vi "RedPitaya_Online_Template_15.12.2019.vi"() -> ()   [LabVIEW 2019]
uses:
  <vilib>/express/express analysis/Spectral/Block/exnSpectralBlock spectral measurements RMS poly.vi
  <vilib>/express/express analysis/Spectral/Block/exnSpectralBlock spectral measurements RMS WFM.vi
  <vilib>/express/express analysis/Spectral/XNode/ExpressSpectralMeasurementsBlockNode.xnode
  <vilib>/Analysis/NI_AAL_SigProc.lvlib
panel:
  in  "Tab Control":T1(tab)
  out "Sensor Signal":sgl[](graph)
  out "Distance [cm]":dbl=113.44243982344857 min=3.0
  out "Location Peaks":dbl[](array[numeric])=[13266.880953082853, 13315.264704454277, 13363.166666666666, 13411.245095976436, 13459.362746922821, 13507.676470231214, 13555.816666494702, 13604.136361362456, 13652.515151704645, 13700.888889844256, 13749.236109598463, 13794.643617108855]
  in  "Peak Threshold":dbl=0.13000000000000012 format="%.2p"
  in  "Sample Threshold":dbl=3000.0 min=3.0
  out "Amplitude Peaks":dbl[](array[numeric])=[1.0525538402918093, 1.1717175096273422, 1.1765014380216599, 1.1719160825014114, 1.1779817342758179, 1.171861931681633, 1.1780178397893906, 1.1718258261680603, 1.1793176233768463, 1.1717897206544876, 1.1821699291467667, 1.171753615140915, 1.184318169951439, 1.1717175096273422, 1.184877797961235, 0.2751458230614705, 1.2100610807538033, 1.1757071167230606, 1.1717175096273422, 1.1720785647630692, 1.1717897206544876, 1.1726201325654984, 1.1720424592494965, 1.176952749490738, 1.1717355698347092, 1.1719521880149841, 1.1719341427087784, 1.175887644290924, 1.1720063537359238, 1.175887644290924, 1.1719521880149841, 1.1751294434070587, 1.1744976043701172, 1.1717716753482819, 1.1717355698347092, 1.1721507757902145, 1.1720063537359238, 1.1727104038000107, 1.1718799769878387, 1.1756890714168549, 1.174901516355678, 1.183162808418274, 1.1716994643211365, 1.1723674088716507, 1.1719521880149841, 1.179714784026146, 1.1716994643211365, 1.1745517551898956, 1.1716994643211365, 1.1733061373233795, 0.621755089566972, 1.171753615140915, 1.1721688210964203, 1.1718258261680603, 1.1855638027191162, 1.1717716753482819, 1.1846972852945328, 1.1933805495500565, 0.9840829961703802, 1.1724576652050018, 1.1742448657751083, 1.1717175096273422, 1.1726381927728653, 1.1718258261680603, 1.1718980371952057, 0.8991820326853672, 0.7123355711971745, 0.3907966132539536, 1.1765375286340714, 1.171970248222351, 1.1716994643211365, 1.1724215596914291, 1.178090050816536, 0.3379421334707791, 0.41264586022121436, 0.14170301344722616, 0.20441930856339144, 0.41122105244403157, 0.1451181683245933, 1.1752962568619767, 1.1743932708955653, 0.956895586745178, 0.2873700125650926, 0.28453465125330124, 0.26024648196001854, 0.22424643172903463, 0.6516108880722223, 0.817807705048344, 0.5987461978823481, 0.20632089172380855, 0.25759756730662464, 0.15722954373967912, 0.39842245914885255, 0.36020466908620663, 0.5011447501881409, 0.40714744730665786, 0.1459626532326326, 0.2610490028596834, 0.2839160048124498, 0.35683245600389685, 0.24854815198521266, 0.21553977557609758, 0.2300543925862896, 0.1404111949016048, 0.13827568641129184, 0.13304504905583056, 0.1480522338098214, 0.20328529691485017, 0.2699936317900817, 0.33758691614384295, 0.39605161937521344, 0.4480722795488725, 0.4914632839585345, 0.5273669232145075, 0.5538165781670914, 0.5719683082015473, 0.5797038517122126, 0.5348972490031214]
  out "Peaks Detected":i32=118
  in  "Width":i32=3 min=3
  in  "Peaks/Valleys":enum32{"Peaks", "Valleys"}(ring)
  out "Reflection":sgl[](graph)=[-0.027295426, -0.027728686, -0.028017526, -0.027439846, -0.027873106, -0.028306367, -0.028595207, -0.028450787, -0.029028468, -0.028884048, -0.027439846, -0.027584266, -0.027728686, -0.027584266, -0.027295426, -0.028161947, -0.027728686, -0.027873106, -0.027728686, -0.027295426, -0.026862165, -0.027151005, -0.028306367, -0.028595207, -0.029172888, -0.028595207, -0.027728686, -0.027439846, -0.027439846, -0.027295426, -0.027295426, -0.027584266, -0.028017526, -0.028306367, -0.029028468, -0.028884048, -0.028161947, -0.028450787, -0.028884048, -0.028884048, -0.028739627, -0.028450787, -0.028306367, -0.028595207, -0.027873106, -0.028017526, -0.028017526, -0.027728686, -0.028884048, -0.029606149, -0.029317308, -0.028161947, -0.027584266, -0.027584266, -0.028450787, -0.028450787, -0.027728686, -0.028161947, -0.028017526, -0.027584266, -0.028161947, -0.027439846, -0.027151005, -0.027584266, -0.027873106, -0.027728686, -0.028017526, -0.028739627, -0.028161947, -0.027873106, -0.028017526, -0.027584266, -0.027295426, -0.027439846, -0.027728686, -0.028450787, -0.028017526, -0.028450787, -0.027873106, -0.027728686, -0.027439846, -0.027728686, -0.028017526, -0.028017526, -0.028884048, -0.028739627, -0.028739627, -0.028595207, -0.028739627, -0.029028468, -0.028739627, -0.028306367, -0.028306367, -0.028739627, -0.028884048, -0.028595207, -0.028595207, -0.028595207, -0.027151005, -0.027728686, -0.028306367, -0.028595207, -0.027873106, -0.028161947, -0.028017526, -0.027584266, -0.028595207, -0.028595207, -0.027728686, -0.027873106, -0.027295426, -0.027728686, -0.028161947, -0.027873106, -0.027873106, -0.027584266, -0.027873106, -0.027439846, -0.027439846, -0.027873106, -0.027295426, -0.026573325, -0.027006585, -0.028161947, -0.028017526, -0.028306367, -0.029317308, -0.027728686, -0.027873106, -0.027584266, -0.028306367, -0.028161947, -0.028884048, -0.029750569, -0.028595207, -0.028739627, -0.028884048, -0.028161947, -0.027728686, -0.027439846, -0.027728686, -0.027873106, -0.028450787, -0.028739627, -0.029028468, -0.029461728, -0.029028468, -0.028161947, -0.027584266, -0.026573325, -0.027584266, -0.028450787, -0.028450787, -0.027873106, -0.028161947, -0.028017526, -0.027584266, -0.027584266, -0.027006585, -0.026140064, -0.026573325, -0.026862165, -0.027295426, -0.027151005, -0.027295426, -0.028017526, -0.028161947, -0.028017526, -0.027873106, -0.028450787, -0.028739627, -0.028739627, -0.029461728, -0.029172888, -0.028450787, -0.029028468, -0.03003941, -0.03047267, -0.03047267, -0.029750569, -0.028450787, -0.028161947, -0.028739627, -0.028017526, -0.028161947, -0.028161947, -0.028017526, -0.027728686, -0.027006585, -0.026862165, -0.027006585, -0.027295426, -0.027151005, -0.026140064, -0.026284484, -0.026573325, -0.026284484, -0.025562381, -0.0249847, -0.0249847, -0.02484028, -0.025851222, -0.025851222, -0.026140064, -0.026428904, -0.026140064, -0.026573325, -0.027584266, -0.028161947, -0.028017526, -0.028595207, -0.029606149, -0.029606149, -0.03133919, -0.031772453, -0.031483613, -0.03191687, -0.032205712, -0.032638974, -0.032494552, -0.032205712, -0.032350134, -0.031772453, -0.03090593, -0.03090593, -0.029606149, -0.028739627, -0.028595207, -0.028450787, -0.027151005, -0.026140064, -0.0249847, -0.023540499, -0.022673978, -0.021518616, -0.020796515, -0.019641152, -0.01906347, -0.019207891, -0.019641152, -0.019785572, -0.019207891, -0.019352311, -0.020218834, -0.020363254, -0.021374196, -0.022673978, -0.02397376, -0.025562381, -0.027584266, -0.029028468, -0.029750569, -0.03133919, -0.033505496, -0.034660857, -0.03538296, -0.03653832, -0.036827162, -0.037404843, -0.038704623, -0.039426725, -0.039426725, -0.040148824, -0.04043767, -0.039859984, -0.038849045, -0.03812694, -0.03697158, -0.035238538, -0.033794336, -0.032205712, -0.03003941, -0.028161947, -0.025562381, -0.022385137, -0.020074412, -0.016897168, -0.014586444, -0.013575503, -0.013142242, -0.010542678, -0.0088096345, -0.007221012, -0.0069321715, -0.0064989105, -0.00621007, -0.0064989105, -0.007943113, -0.009676156, -0.01242014, -0.014586444, -0.017474849, -0.020218834, -0.023684919, -0.026428904, -0.029750569, -0.033361074, -0.03668274, -0.039426725, -0.04245955, -0.044914693, -0.04794752, -0.050691504, -0.053002227, -0.055457372, -0.056323893, -0.05589063, -0.05617947, -0.05589063, -0.055457372, -0.05430201, -0.051558025, -0.04910288, -0.044481434, -0.040582087, -0.03697158, -0.032638974, -0.028161947, -0.02397376, -0.01906347, -0.012997821, -0.0077986927, -0.0037549261, 0.00043326072, 0.0040437668, 0.0067877513, 0.009242895, 0.011698039, 0.013719923, 0.013864343, 0.01242014, 0.010975938, 0.009242895, 0.0070765917, 0.003610506, -0.00086652144, -0.005343549, -0.010831518, -0.016463907, -0.022240717, -0.027873106, -0.034516435, -0.04043767, -0.046214476, -0.051991284, -0.057334833, -0.063400485, -0.06802193, -0.07293222, -0.07654273, -0.07842019, -0.080730915, -0.08145302, -0.08000881, -0.07899787, -0.076831564, -0.07452084, -0.069899395, -0.06426701, -0.058634616, -0.051558025, -0.045059115, -0.037116002, -0.029028468, -0.020796515, -0.012997821, -0.0056323893, 0.0027439846, 0.010542678, 0.016897168, 0.022673978, 0.028306367, 0.032494552, 0.03538296, 0.03697158, 0.037982523, 0.037693683, 0.035238538, 0.032494552, 0.028161947, 0.022818398, 0.015741806, 0.010253837, 0.0023107238, -0.0056323893, -0.014586444, -0.02397376, -0.034083176, -0.044192594, -0.053579908, -0.06253396, -0.07105476, -0.07914229, -0.0870854, -0.09343989, -0.099072285, -0.10239395, -0.10542677, -0.108170755, -0.1091817, -0.107159816, -0.10369373, -0.09878344, -0.092573375, -0.08593004, -0.07755367, -0.06917729, -0.058056936, -0.04809194, -0.037116002, -0.025273541, -0.013864343, -0.002455144, 0.008665214, 0.019496731, 0.03003941, 0.039571144, 0.04751426, 0.05415759, 0.059501138, 0.062822804, 0.06542237, 0.06672215, 0.06571121, 0.06311164, 0.058345776, 0.052713387, 0.045347955, 0.036827162, 0.027006585, 0.016463907, 0.0046214475, -0.0064989105, -0.01891905, -0.032494552, -0.0463589, -0.06094534, -0.07437642, -0.08679657, -0.09820576, -0.108748436, -0.11755808, -0.12535676, -0.13171126, -0.13589944, -0.13821016, -0.13821016, -0.13676597, -0.13329989, -0.12867843, -0.122323945, -0.113514304, -0.10354931, -0.09228453, -0.07943113, -0.065566786, -0.050980344, -0.03480528, -0.017474849, -0.0012997822, 0.013864343, 0.028739627, 0.04245955, 0.05560179, 0.06816635, 0.07856461, 0.088240765, 0.095172934, 0.0999388, 0.102249525, 0.10311605, 0.101671845, 0.09748366, 0.09112917, 0.082897216, 0.07264338, 0.06123418, 0.04765868, 0.032927815, 0.015886227, -0.0014442024, -0.019785572, -0.0378381, -0.055746213, -0.07379874, -0.09343989, -0.109903805, -0.12521234, -0.13878785, -0.1499082, -0.16016205, -0.16868284, -0.1748929, -0.17835899, -0.1798032, -0.17807016, -0.17330429, -0.16651653, -0.1569848, -0.14586444, -0.1320001, -0.11568061, -0.09791692, -0.07928671, -0.05935672, -0.038271364, -0.017041588, 0.004910288, 0.025706802, 0.045059115, 0.06383374, 0.082319535, 0.09863903, 0.113514304, 0.12550119, 0.13546619, 0.1426872, 0.14687538, 0.14803074, 0.14615329, 0.14080973, 0.13243335, 0.12189068, 0.10961496, 0.093151055, 0.074809685, 0.05560179, 0.034372017, 0.011409199, -0.011264779, -0.0363939, -0.062245123, -0.0870854, -0.10932612, -0.1320001, -0.1535187, -0.17214893, -0.18861283, -0.20233275, -0.2147529, -0.22298485, -0.22789514, -0.23006144, -0.22789514, -0.22298485, -0.21489732, -0.20305486, -0.18861283, -0.1698382, -0.14947495, -0.12622328, -0.101238586, -0.07553179, -0.04823636, -0.020652095, 0.0063544903, 0.033505496, 0.06181186, 0.088818446, 0.11380315, 0.13575502, 0.15496291, 0.17186008, 0.18529117, 0.19511174, 0.20132181, 0.20319928, 0.2026216, 0.19785573, 0.18731305, 0.17431523, 0.15814017, 0.13792133, 0.11481409, 0.08896287, 0.06051208, 0.03105035, 0.00014442024, -0.032061294, -0.064411424, -0.09820576, -0.12968938, -0.1591511, -0.18615769, -0.21186449, -0.23482731, -0.25360194, -0.2690549, -0.28104177, -0.28941816, -0.292451, -0.2905735, -0.28494114, -0.27454287, -0.25880107, -0.2404597, -0.21821898, -0.19222334, -0.16348371, -0.13185568, -0.09835018, -0.06311164, -0.026284484, 0.010253837, 0.04722542, 0.08304164, 0.11596945, 0.1477419, 0.17734805, 0.20392138, 0.22544, 0.24349253, 0.25721243, 0.26645535, 0.26992142, 0.2681884, 0.2618339, 0.24984701, 0.23352753, 0.21287543, 0.18803515, 0.15900669, 0.12737866, 0.09185127, 0.05372433, 0.013719923, -0.028450787, -0.069899395, -0.11105917, -0.15005262, -0.18817957, -0.22471789, -0.25750127, -0.2853744, -0.3103591, -0.33043352, -0.3454532, -0.35498494, -0.35873988, -0.35772893, -0.3503635, -0.3375101, -0.31945756, -0.29707244, -0.2691993, -0.23742688, -0.20103297, -0.16117299, -0.119002275, -0.07610947, -0.03133919, 0.014297604, 0.06022324, 0.10470467, 0.14730865, 0.18687978, 0.22226274, 0.25287983, 0.28104177, 0.30342692, 0.3197464, 0.3318777, 0.3373657, 0.3354882, 0.32725626, 0.31295866, 0.29317307, 0.2690549, 0.23887107, 0.20305486, 0.16333929, 0.12044648, 0.07466526, 0.026717745, -0.023251658, -0.074232005, -0.12304604, -0.17027146, -0.21663035, -0.25923434, -0.29808336, -0.33346632, -0.36379457, -0.3873351, -0.40495434, -0.4175189, -0.42358455, -0.42214036, -0.4140528, -0.39903313, -0.37852544, -0.3518077, -0.3190243, -0.2804641, -0.2375713, -0.19077913, -0.14182067, -0.09084033, -0.03754926, 0.016319487, 0.07004382, 0.12030206, 0.16998263, 0.21648593, 0.25952315, 0.2982278, 0.32985583, 0.35556263, 0.37549263, 0.38921255, 0.39556703, 0.3945561, 0.38632414, 0.37101558, 0.34906372, 0.32075736, 0.28638533, 0.2462365, 0.2004553, 0.15048589, 0.09748366, 0.04231513, -0.014297604, -0.07192128, -0.12766749, -0.18240276, -0.23540498, -0.28522998, -0.3311556, -0.37217095, -0.40668738, -0.43571585, -0.458101, -0.47254303, -0.4788975, -0.47788656, -0.4689325, -0.4531907, -0.4303723, -0.40047732, -0.3632169, -0.32003525, -0.272521, -0.22226274, -0.16810516, -0.10961496, -0.050691504, 0.010253837, 0.07119918, 0.12867843, 0.18456906, 0.23699361, 0.28494114, 0.32855603, 0.36668298, 0.39773333, 0.4211294, 0.43730447, 0.44582528, 0.4475583, 0.4394708, 0.42358455, 0.39946637, 0.36942697, 0.33231097, 0.28884047, 0.23915991, 0.18558, 0.12795633, 0.06672215, 0.004188187, -0.05877904, -0.12304604, -0.18370254, -0.2433481, -0.30024967, -0.35281864, -0.39859986, -0.43802658, -0.47052112, -0.49651676, -0.5147137, -0.52568966, -0.5284337, -0.5216459, -0.5066262, -0.482508, -0.45073557, -0.41260862, -0.36668298, -0.3154138, -0.25923434, -0.19944435, -0.13618828, -0.07119918, -0.0056323893, 0.06094534, 0.124923505, 0.18716863, 0.24681419, 0.30198273, 0.34993023, 0.39311188, 0.42849484, 0.45622352, 0.47702006, 0.48857367, 0.49131766, 0.48539641, 0.4709544, 0.44856927, 0.41708565, 0.37866986, 0.33288866, 0.28075296, 0.22356252, 0.16189508, 0.09676156, 0.029750569, -0.039137885, -0.1084596, -0.17518175, -0.24074854, -0.30357134, -0.36047292, -0.41231978, -0.45795658, -0.49651676, -0.5274227, -0.5500967, -0.5632389, -0.56713825, -0.56266123, -0.549519, -0.52814484, -0.4968056, -0.45781216, -0.4118865, -0.3581622, -0.29938316, -0.2361271, -0.16882727, -0.0999388, -0.029317308, 0.04260397, 0.112503365, 0.18009204, 0.24450347, 0.3048711, 0.3597508, 0.4087093, 0.4495802, 0.48178592, 0.5059041, 0.52121264, 0.5272783, 0.5238122, 0.51196975, 0.49073997, 0.45983404, 0.4211294, 0.37592587, 0.3224904, 0.26313367, 0.19843341, 0.13026705, 0.059212297, -0.013142242, -0.087663084, -0.15929553, -0.22991702, -0.29736128, -0.35989523, -0.41694123, -0.46792158, -0.5109588, -0.5459085, -0.57277066, -0.591112, -0.5997772, -0.59818864, -0.58692384, -0.5662718, -0.53551024, -0.49767214, -0.45116884, -0.3975889, -0.33765453, -0.27223215, -0.20291044, -0.12968938, -0.05516853, 0.01877463, 0.093728736, 0.16593885, 0.23468289, 0.29996082, 0.35902873, 0.41203094, 0.4573789, 0.4946393, 0.5229457, 0.5427312, 0.5525518, 0.5526962, 0.5433089, 0.524101, 0.49536142, 0.458101, 0.4124642, 0.35946196, 0.299672, 0.23482731, 0.16463907, 0.09141801, 0.016030647, -0.06007882, -0.13662155, -0.21114239, -0.2832081, -0.35094118, -0.4124642, -0.4673439, -0.51442486, -0.5544293, -0.5859129, -0.6071427, -0.6184075, -0.621007, -0.61320835, -0.5951558, -0.5675715, -0.5310332, -0.4859741, -0.43282744, -0.3731819, -0.30862606, -0.23742688, -0.16247277, -0.086074464, -0.009387315, 0.06859961, 0.14369814, 0.2176413, 0.28667417, 0.3497858, 0.40654296, 0.45607913, 0.49752772, 0.5307444, 0.5542849, 0.56786036, 0.5719041, 0.5655497, 0.54908574, 0.52251244, 0.4881404, 0.4438034, 0.39224535, 0.3338996, 0.26862165, 0.19814457, 0.12304604, 0.046792157, -0.031483613, -0.110481486, -0.18731305, -0.2619783, -0.33259982, -0.39787775, -0.45636794, -0.5073483, -0.55168533, -0.5875015, -0.61306393, -0.6289501, -0.6344381, -0.6295278, -0.6145081, -0.5901011, -0.55674005, -0.5142805, -0.4630113, -0.40394342, -0.33794335, -0.267033, -0.19308986, -0.116980396, -0.038849045, 0.04072651, 0.11856902, 0.19366755, 0.26529998, 0.33216655, 0.39238977, 0.44640297, 0.4916065, 0.5277116, 0.55414045, 0.5717597, 0.579414, 0.57667, 0.56338334, 0.54056495, 0.5086481, 0.46705505, 0.4167968, 0.36003965, 0.29562822, 0.22500673, 0.15164125, 0.07408758, -0.004332607, -0.08376374, -0.16088414, -0.23742688, -0.30949256, -0.37708125, -0.4388931, -0.49348396, -0.5408538, -0.5792696, -0.6080092, -0.62692827, -0.6355935, -0.6338604, -0.6228845, -0.602088, -0.5706044, -0.5301667, -0.48135266, -0.4245955, -0.36148384, -0.29259542, -0.22038528, -0.14427581, -0.06600005, 0.012997821, 0.09141801, 0.16738306, 0.2397376, 0.30790395, 0.37072676, 0.42632854, 0.47355396, 0.512403, 0.5280004, 0.43499374, 0.34559762, 0.27959758, 0.22933933, 0.19020145, 0.15727364, 0.12925611, 0.10586003, 0.083908156, 0.06311164, 0.04274839, 0.022529557, 0.0021663036, -0.01776369, -0.037693683, -0.057190415, -0.07827577, -0.10326047, -0.115825035, -0.1283896, -0.13979879, -0.15019704, -0.15972878, -0.16680537, -0.17171566, -0.17431523, -0.17518175, -0.17373754, -0.16853842, -0.16102856, -0.15164125, -0.14037648, -0.12622328, -0.110914744, -0.09502852, -0.07813135, -0.0599344, -0.04159303, -0.022529557, -0.0025995644, 0.015164125, 0.032638974, 0.049824983, 0.06513353, 0.08694098, 0.09748366, 0.10412699, 0.10975938, 0.11380315, 0.11654713, 0.11669155, 0.11481409, 0.1106259, 0.10369373, 0.09546178, 0.084197, 0.070477076, 0.056035053, 0.040293247, 0.023107238, 0.0056323893, -0.01242014, -0.03076151, -0.050113823, -0.06816635, -0.09228453, -0.10975938, -0.122757204, -0.1334443, -0.14413139, -0.1535187, -0.16001762, -0.16565001, -0.16882727, -0.17012703, -0.16940494, -0.16536117, -0.15900669, -0.15048589, -0.14052089, -0.12810075, -0.11438083, -0.09878344, -0.0820307, -0.064411424, -0.046503317, -0.028739627, -0.010831518, 0.0075098523, 0.02484028, 0.041448608, 0.056612734, 0.0713436, 0.090407066, 0.0970504, 0.10239395, 0.10744866, 0.11077032, 0.111348, 0.11004822, 0.106148876, 0.100083224, 0.091995694, 0.08217511, 0.07076592, 0.057768095, 0.04318165, 0.027728686, 0.010542678, -0.0069321715, -0.02512912, -0.043037232, -0.06108976, -0.08000881, -0.10268279, -0.11322547, -0.124345824, -0.13561061, -0.1448535, -0.15308546, -0.15900669, -0.16218393, -0.16362813, -0.16377255, -0.16045089, -0.15539618, -0.14788632, -0.13878785, -0.12824517, -0.11568061, -0.10152743, -0.08621888, -0.06946614, -0.051991284, -0.034516435, -0.017186008, -0.00086652144, 0.015741806, 0.031483613, 0.0463589, 0.06036766, 0.07654273, 0.088818446, 0.094161995, 0.09878344, 0.102249525, 0.10412699, 0.10297163, 0.10022765, 0.0948841, 0.08838519, 0.080153234, 0.06975497, 0.057623673, 0.044192594, 0.029461728, 0.014008763, -0.0014442024, -0.01776369, -0.0356718, -0.05256897, -0.06859961, -0.09011823, -0.10484909, -0.11524735, -0.12535676, -0.1348885, -0.14297603, -0.14860843, -0.15250777, -0.15467407, -0.15510733, -0.1535187, -0.14904168, -0.14254278, -0.13445525, -0.12506792, -0.11423641, -0.101238586, -0.08751866, -0.07235454, -0.05617947, -0.04043767, -0.02469586, -0.008665214, 0.0069321715, 0.022240717, 0.03726042, 0.05025824, 0.06152302, 0.076398306, 0.08737425, 0.09069591, 0.093584314, 0.09459525, 0.09445084, 0.09286221, 0.08896287, 0.083908156, 0.07668715, 0.06744425, 0.056323893, 0.044192594, 0.03032825, 0.016463907, 0.0011553619, -0.015164125, -0.03119477, -0.046214476, -0.06094534, -0.075820625, -0.098494604, -0.10730424, -0.116402715, -0.1242014, -0.13171126, -0.13806574, -0.14297603, -0.14514235, -0.14543118, -0.14470908, -0.14210951, -0.13676597, -0.13041148, -0.122323945, -0.11221453, -0.10051648, -0.08694098, -0.07307664, -0.05877904, -0.044192594, -0.029028468, -0.013864343, 0.00086652144, 0.014442024, 0.027295426, 0.039715566, 0.05025824, 0.06080092, 0.07235454, 0.083908156, 0.08448584, 0.0856412, 0.08621888, 0.08434142, 0.08159743, 0.07755367, 0.070332654, 0.062245123, 0.05314665, 0.04217071, 0.029894989, 0.015886227, 0.0028884048, -0.0111203585, -0.025562381, -0.040148824, -0.05444643, -0.06744425, -0.084197, -0.100660905, -0.10802634, -0.11481409, -0.121168576, -0.12694539, -0.13142242, -0.13474408, -0.13546619, -0.13532177, -0.1327222, -0.12896727, -0.12362372, -0.115825035, -0.10687098, -0.09661714, -0.08549678, -0.07408758, -0.0606565, -0.04693658, -0.033361074, -0.019496731, -0.0067877513, 0.00606565, 0.01805253, 0.029461728, 0.040582087, 0.049824983, 0.057912517, 0.064411424, 0.074809685, 0.08058649, 0.07813135, 0.07610947, 0.0735099, 0.06917729, 0.062822804, 0.055457372, 0.046792157, 0.03812694, 0.027584266, 0.016319487, 0.0038993463, -0.009387315, -0.022096297, -0.03480528, -0.04751426, -0.06007882, -0.07177686, -0.08968497, -0.09921671, -0.10513794, -0.110914744, -0.115825035, -0.120013215, -0.12304604, -0.12463467, -0.12506792, -0.12347931, -0.12073532, -0.115825035, -0.10975938, -0.101671845, -0.09329548, -0.0834749, -0.07192128, -0.06022324, -0.0485252, -0.03581622, -0.023107238, -0.0111203585, 0.00057768094, 0.011264779, 0.021374196, 0.03119477, 0.040004406, 0.047080997, 0.05285781, 0.057479255, 0.061378602, 0.06325606, 0.062967226, 0.061667442, 0.058923457, 0.05487969, 0.04895846, 0.04245955, 0.033649914, 0.02455144, 0.014153183, 0.0038993463, -0.007365432, -0.019207891, -0.03076151, -0.04188187, -0.053002227, -0.06412259, -0.07466526, -0.0834749, -0.09214011, -0.09892786, -0.10513794, -0.10932612, -0.11178126, -0.11336989, -0.114091985, -0.113514304, -0.111348, -0.10672656, -0.10138301, -0.095172934, -0.08751866, -0.07943113, -0.070332654, -0.06080092, -0.05025824, -0.039137885, -0.027873106, -0.017186008, -0.0070765917, 0.003610506, 0.013286662, 0.022385137, 0.03047267, 0.037116002, 0.04274839, 0.04693658, 0.050691504, 0.052280128, 0.053002227, 0.052280128, 0.050113823, 0.046503317, 0.04217071, 0.03610506, 0.029894989, 0.021951877, 0.012853401, 0.0033216656, -0.0067877513, -0.017330429, -0.027584266, -0.03754926, -0.04765868, -0.057479255, -0.06672215, -0.074809685, -0.082319535, -0.08838519, -0.09430642, -0.09878344, -0.10210511, -0.10398257, -0.10427141, -0.10354931, -0.10152743, -0.09892786, -0.09430642, -0.08852961, -0.08188628, -0.074809685, -0.06686657, -0.057623673, -0.04809194, -0.039282303, -0.03032825, -0.020796515, -0.011553619, -0.002455144, 0.0063544903, 0.014008763, 0.020796515, 0.027006585, 0.032205712, 0.03610506, 0.038704623, 0.04101535, 0.04260397, 0.04274839, 0.04072651, 0.03726042, 0.032350134, 0.027873106, 0.022385137, 0.015597385, 0.008520794, 0.0010109417, -0.0077986927, -0.016752748, -0.025706802, -0.034660857, -0.04318165, -0.051413603, -0.05935672, -0.06686657, -0.0735099, -0.07957555, -0.0849191, -0.088818446, -0.09112917, -0.09286221, -0.09343989, -0.09343989, -0.09185127, -0.08896287, -0.08621888, -0.08145302, -0.07654273, -0.07018824, -0.062822804, -0.05502411, -0.04722542, -0.039426725, -0.031483613, -0.022962818, -0.015019705, -0.007943113, -0.00086652144, 0.006643331, 0.012853401, 0.01819695, 0.023251658, 0.027295426, 0.03003941, 0.031772453, 0.03191687, 0.03191687, 0.03105035, 0.028739627, 0.025273541, 0.021229776, 0.015597385, 0.0103982575, 0.0046214475, -0.0021663036, -0.009387315, -0.016897168, -0.02469586, -0.032205712, -0.040004406, -0.047369838, -0.05415759, -0.06094534, -0.06628889, -0.07105476, -0.075387366, -0.07870903, -0.081308596, -0.08304164, -0.084197, -0.08405258, -0.082897216, -0.080730915, -0.07769809, -0.07408758, -0.070332654, -0.06513353, -0.058634616, -0.052135706, -0.045636795, -0.039282303, -0.032350134, -0.025706802, -0.01863021, -0.011409199, -0.0051991288, 0.00057768094, 0.0057768095, 0.009964996, 0.014153183, 0.01776369, 0.020363254, 0.022673978, 0.023107238, 0.023107238, 0.021951877, 0.020507675, 0.017474849, 0.0134310825, 0.009387315, 0.0046214475, -0.00028884047, -0.005343549, -0.011409199, -0.01819695, -0.02469586, -0.03076151, -0.036827162, -0.04347049, -0.049247302, -0.05473527, -0.05964556, -0.06412259, -0.06701099, -0.069899395, -0.07249896, -0.074809685, -0.07553179, -0.075242944, -0.07408758, -0.07235454, -0.06961056, -0.06643331, -0.06253396, -0.05906788, -0.05487969, -0.04895846, -0.04375933, -0.037693683, -0.03162803, -0.026428904, -0.020363254, -0.014297604, -0.009676156, -0.004910288, 0.0, 0.004188187, 0.0076542725, 0.010687098, 0.01242014, 0.0134310825, 0.014153183, 0.014008763, 0.013719923, 0.01242014, 0.010253837, 0.007221012, 0.0038993463, -0.00057768094, -0.004910288, -0.0103982575, -0.015452965, -0.020218834, -0.02512912, -0.03018383, -0.03509412, -0.040582087, -0.044914693, -0.049536142, -0.05386875, -0.057334833, -0.06022324, -0.06267838, -0.064555846, -0.06614447, -0.06686657, -0.06672215, -0.06571121, -0.06484469, -0.06311164, -0.06036766, -0.057045992, -0.053002227, -0.04939172, -0.045781214, -0.04101535, -0.03624948, -0.03162803, -0.026428904, -0.021663036, -0.017619269, -0.0134310825, -0.009676156, -0.0056323893, -0.0021663036, 0.0014442024, 0.0034660858, 0.0056323893, 0.0067877513, 0.0069321715, 0.0069321715, 0.0059212297, 0.0038993463, 0.0018774631, -0.00014442024, -0.0027439846, -0.0057768095, -0.009676156, -0.013575503, -0.01805253, -0.021807456, -0.025995642, -0.03003941, -0.034660857, -0.038704623, -0.04260397, -0.045781214, -0.04881404, -0.051558025, -0.05430201, -0.05589063, -0.057190415, -0.058345776, -0.058923457, -0.058634616, -0.058490198, -0.057190415, -0.05560179, -0.05372433, -0.050835922, -0.04794752, -0.045059115, -0.04188187, -0.038271364, -0.034516435, -0.03003941, -0.025851222, -0.022385137, -0.01891905, -0.015308545, -0.011842459, -0.008954055, -0.0064989105, -0.0050547086, -0.003610506, -0.0020218834, -0.0011553619, -0.00043326072, -0.00057768094, -0.0014442024, -0.0021663036, -0.0037549261, -0.0059212297, -0.008231954, -0.010975938, -0.013719923, -0.016319487, -0.019785572, -0.02382934, -0.027728686, -0.03105035, -0.033794336, -0.036827162, -0.039859984, -0.043037232, -0.045925636, -0.04823636, -0.050113823, -0.051124763, -0.051846866, -0.052713387, -0.053002227, -0.05285781, -0.051846866, -0.050691504, -0.049536142, -0.04765868, -0.045347955, -0.043037232, -0.04043767, -0.037693683, -0.034516435, -0.03162803, -0.028739627, -0.026717745, -0.023251658, -0.019785572, -0.017474849, -0.015308545, -0.013142242, -0.011409199, -0.009964996, -0.008231954, -0.007365432, -0.006643331, -0.0063544903, -0.006643331, -0.0069321715, -0.007943113, -0.009676156, -0.010975938, -0.013575503, -0.016319487, -0.01877463, -0.020363254, -0.023107238, -0.025562381, -0.027728686, -0.03047267, -0.033361074, -0.03552738, -0.038271364, -0.040004406, -0.04260397, -0.044337012, -0.045492373, -0.046792157, -0.047080997, -0.046792157, -0.047080997, -0.04664774, -0.045781214, -0.045203533, -0.044192594, -0.04347049, -0.04130419, -0.039426725, -0.036827162, -0.034372017, -0.032205712, -0.029894989, -0.027295426, -0.02455144, -0.022673978, -0.021085355, -0.01877463, -0.017186008, -0.015741806, -0.014586444, -0.0134310825, -0.01242014, -0.011553619, -0.0111203585, -0.011698039, -0.011553619, -0.01242014, -0.013286662, -0.014297604, -0.016030647, -0.017041588, -0.01848579, -0.020652095, -0.023107238, -0.025273541, -0.027584266, -0.029750569, -0.03191687, -0.033938754, -0.03581622, -0.0378381, -0.039137885, -0.04043767, -0.041448608, -0.043037232, -0.04289281, -0.04274839, -0.04375933, -0.04347049, -0.04245955, -0.04159303, -0.040870927, -0.039571144, -0.03812694, -0.03668274, -0.03480528, -0.032494552, -0.03105035, -0.029750569, -0.028161947, -0.026140064, -0.02484028, -0.023107238, -0.021229776, -0.020218834, -0.01891905, -0.017330429, -0.016030647, -0.015308545, -0.014730864, -0.015164125, -0.015452965, -0.015741806, -0.015886227, -0.016608328, -0.01790811, -0.01863021, -0.019641152, -0.020796515, -0.022529557, -0.0249847, -0.025851222, -0.027439846, -0.029461728, -0.03119477, -0.032638974, -0.034227595, -0.034660857, -0.03624948, -0.037116002, -0.03812694, -0.039426725, -0.040148824, -0.040293247, -0.040148824, -0.039715566, -0.039282303, -0.038849045, -0.03812694, -0.03726042, -0.03653832, -0.034949698, -0.032927815, -0.03162803, -0.029606149, -0.028161947, -0.027295426, -0.025417961, -0.0242626, -0.022962818, -0.022096297, -0.021085355, -0.019785572, -0.01863021, -0.01863021, -0.01891905, -0.01891905, -0.01891905, -0.01863021, -0.01863021, -0.01891905, -0.01906347, -0.019207891, -0.020507675, -0.021518616, -0.023251658, -0.02440702, -0.025706802, -0.027295426, -0.028595207, -0.03047267, -0.03162803, -0.032350134, -0.033505496, -0.034516435, -0.03538296, -0.03668274, -0.03668274, -0.037404843, -0.03812694, -0.0378381, -0.037982523, -0.037693683, -0.037116002, -0.0363939, -0.0356718, -0.03480528, -0.033938754, -0.032783393, -0.031483613, -0.03018383, -0.029172888, -0.028017526, -0.027006585, -0.025995642, -0.02455144, -0.023540499, -0.022240717, -0.021374196, -0.021229776, -0.020796515, -0.019929992, -0.019496731, -0.019785572, -0.019641152, -0.020507675, -0.020507675, -0.020363254, -0.021085355, -0.021807456, -0.022818398, -0.023684919, -0.02469586, -0.025851222, -0.027295426, -0.028595207, -0.029894989, -0.03090593, -0.032205712, -0.033216655, -0.034083176, -0.034372017, -0.03480528, -0.0356718, -0.03610506, -0.0356718, -0.03581622, -0.035238538, -0.03581622, -0.03596064, -0.0356718, -0.035238538, -0.034227595, -0.033216655, -0.032205712, -0.03047267, -0.029894989, -0.028595207, -0.028017526, -0.027439846, -0.025995642, -0.02469586, -0.023684919, -0.022818398, -0.022818398]
  in  "Delay (# Samples)":i32=8192 max=100000
  out "Temp [°C]":dbl=23.2051 format="%#_2g"
  out "Samplerate":dbl=1953125.0
  out "Fourier Spectrum":cluster{"f0":dbl, "df":dbl, "magnitude":dbl[]}(graph)={"f0"=0.0, "df"=0.00048828125, "magnitude"=[]}
  in  "Threshold peak detect.":dbl caption="Threshold Peak Detection" format="%0.4f"
  in  "Width peak detect.":i32=4 caption="Width Peak Detection" min=3
  out "# Peaks":i32
  out "SINAD (dB)":dbl
  out "Loc 1st Peak":dbl
  out "Peak to Peak":dbl
  out "Positive Peak":dbl
  out "Negative Peak":dbl
  out "Mean (DC)":dbl
  out "RMS Value":dbl
  in  "Number 1":dbl
  in  "Number 2":dbl
  out "Result":dbl
  out "error out 2":errorcluster
  in  "Host IP address":string="192.168.128.1"
  out "Fehlermeldung":string
  out "Rückgabe":string
  out "Ausgeführter Befehl":string="C:\\Users\\DiSiLabXX\\Desktop\\US_24.10.19\\plink.exe root@192.168.128.1 -ssh -pw root -m \"config.txt\""
  in  "timeout ms (2000)":i32=400
  in  "Stop":bool
  # "Version 05_15.12.19\nFb2/Michalik"
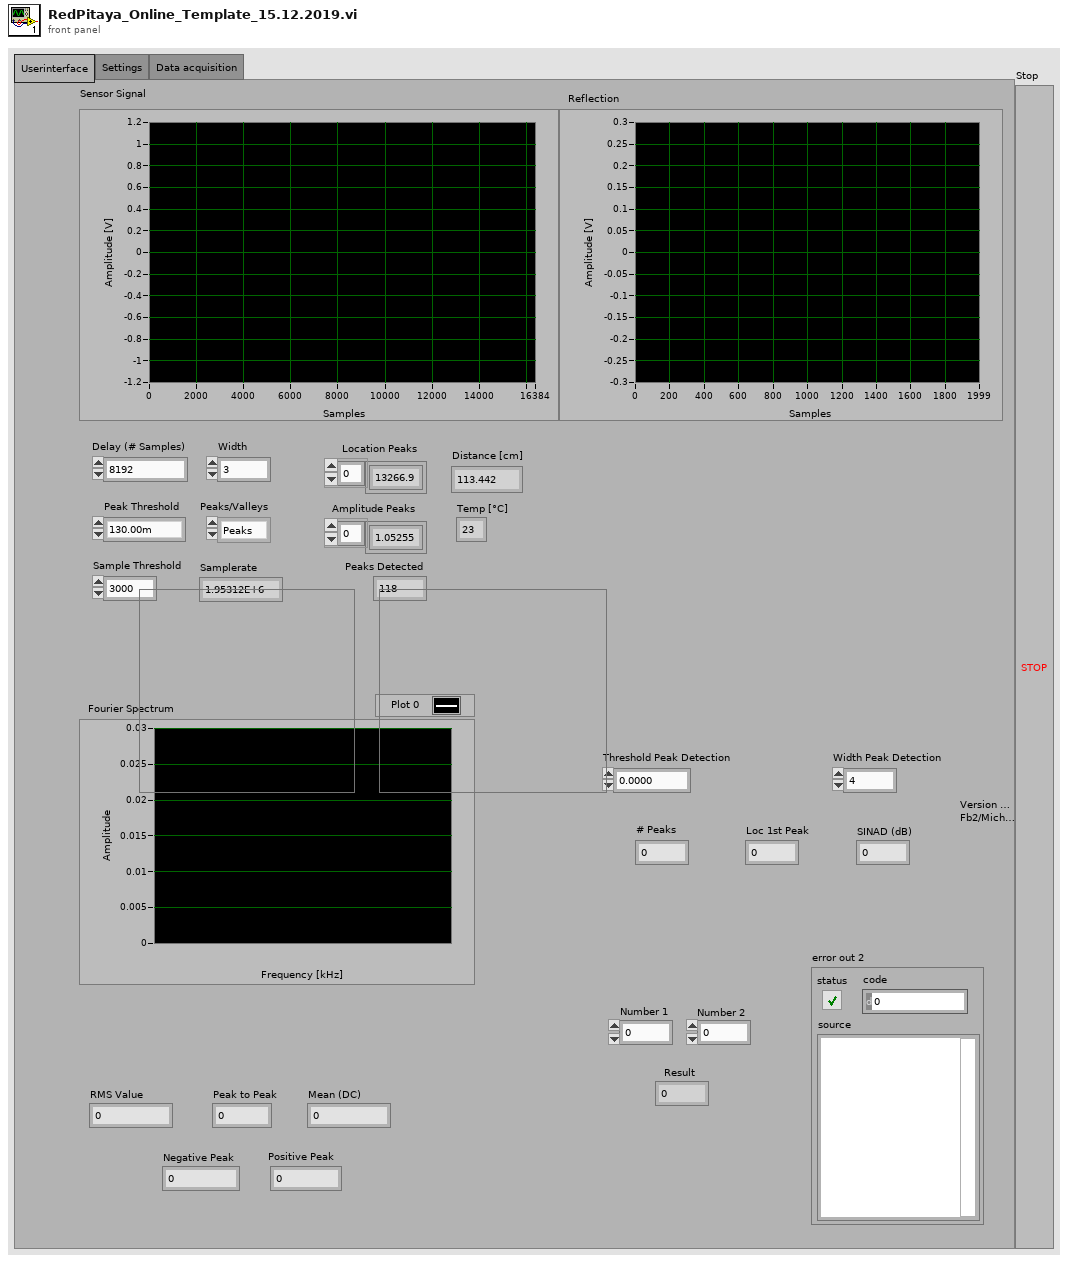
[diagram p1: front panel]
types:
  T1 = enum32{"Userinterface", "Settings", "Data acquisition"}
  T2 = enum16{"Standard", "Buffered", "CRLF", "Immediate"}
  T3 = cluster{"averaging mode":u16, "weighting mode":u16, "number of averages":u32}
  T4 = cluster{"dB On (F)":bool, "unwrap phase (F)":bool, "convert to degree (F)":bool}
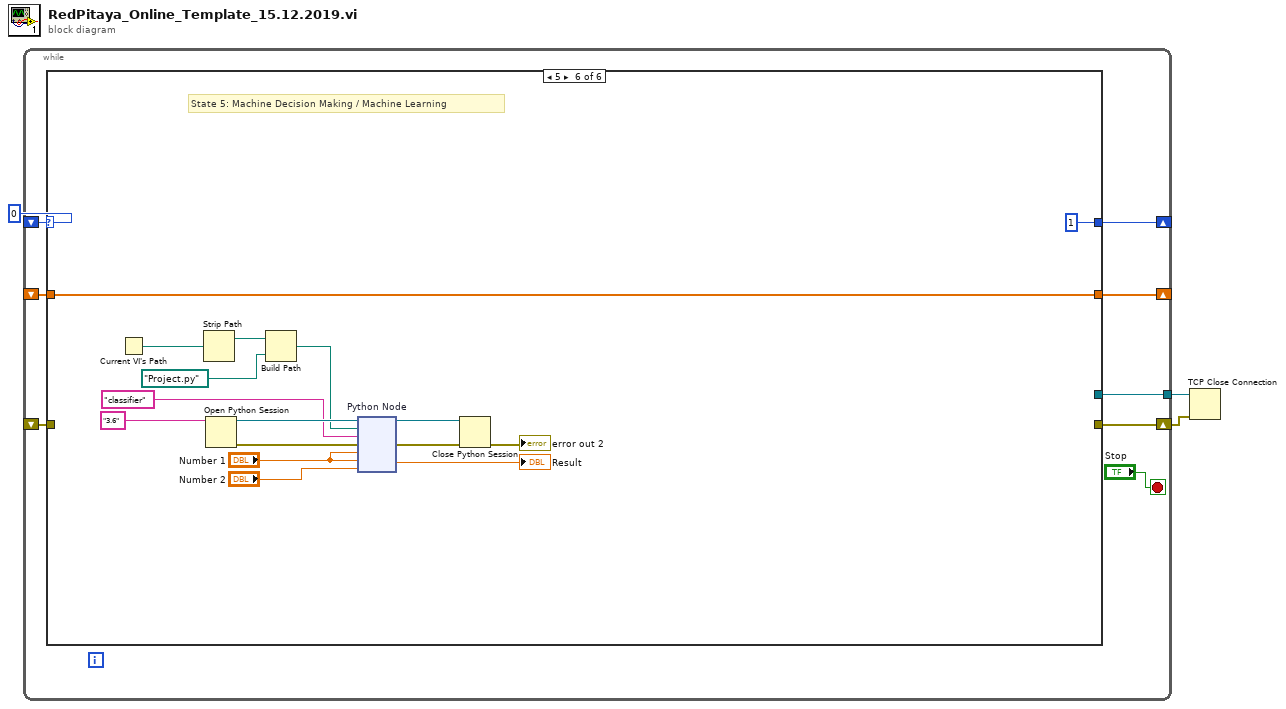
[diagram p0: block diagram]
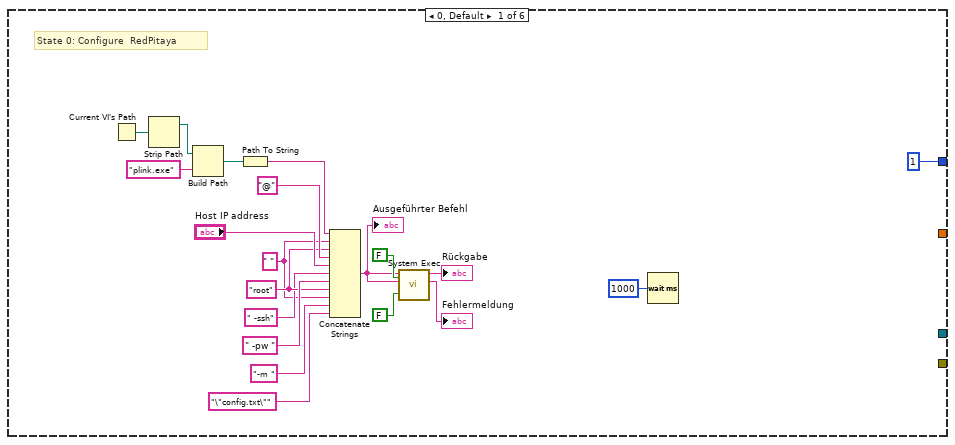
[diagram p2: hidden frame]
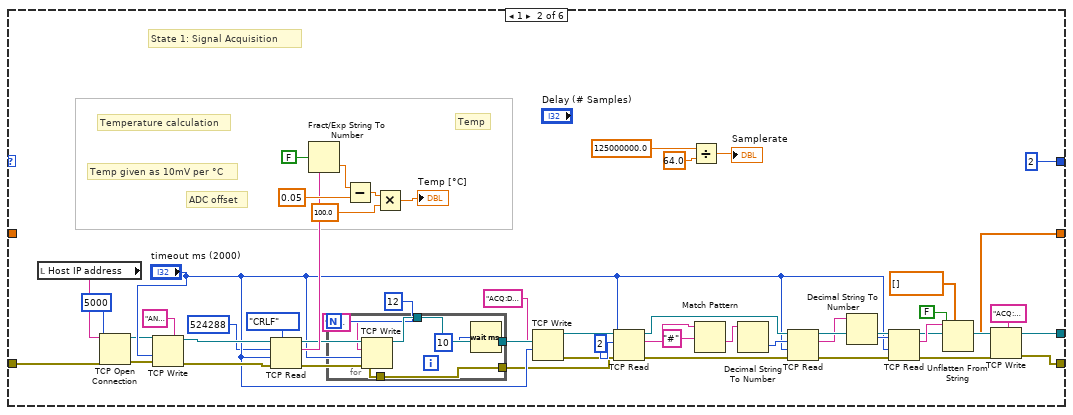
[diagram p3: hidden frame]
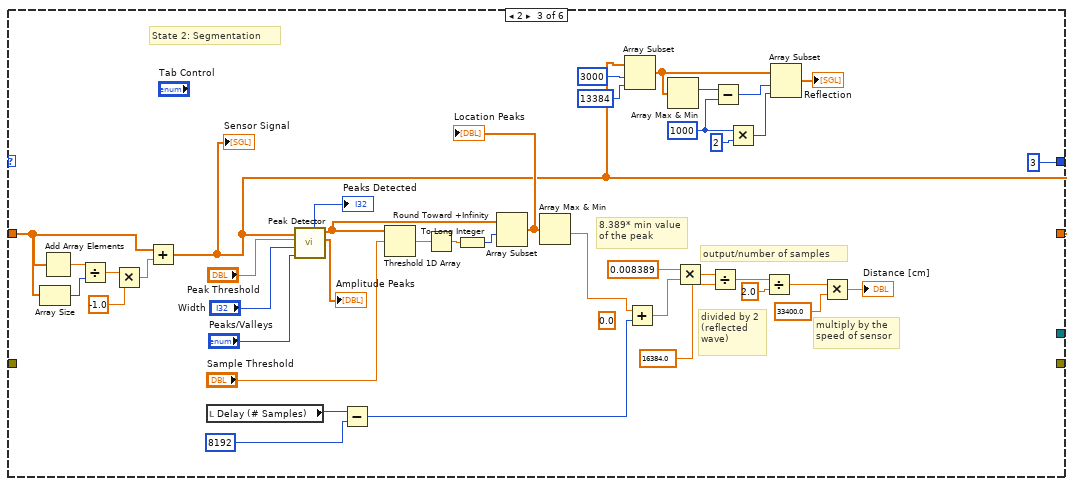
[diagram p4: hidden frame]
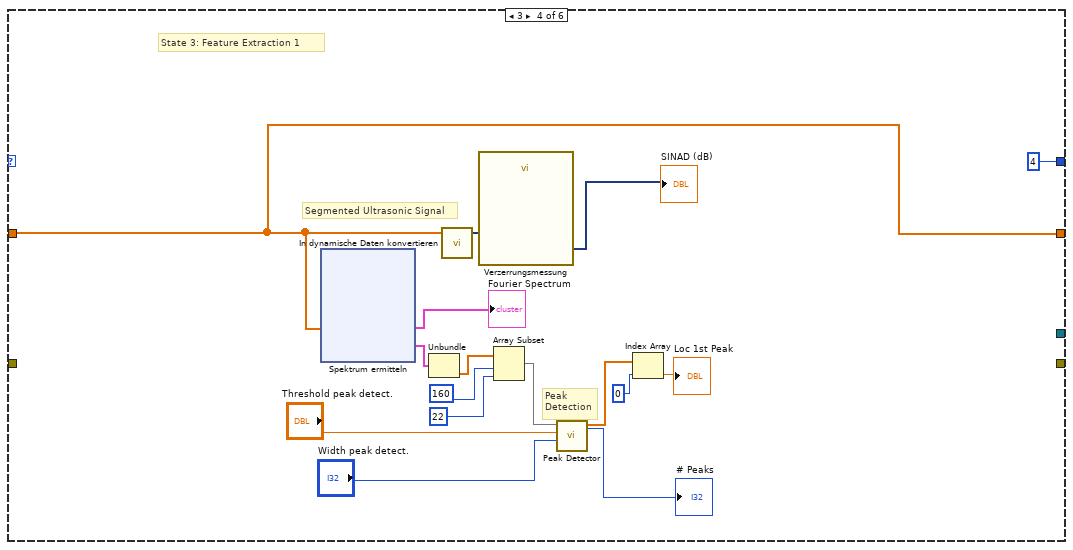
[diagram p5: hidden frame]
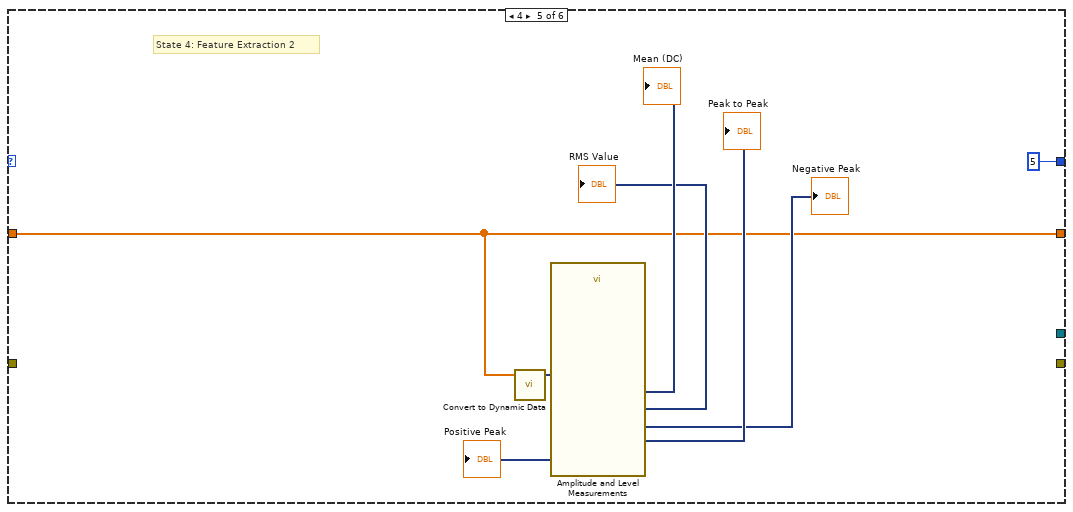
[diagram p6: hidden frame]
diagram:
  n1 = while {
    shift-right: [w10] -> _
    shift-left: 0 -> [w11]
    shift-right: [w8] -> _
    shift-left: _ -> [w7]
    tunnel: [w6] -> w2
    shift-right: [w4] -> w1
    shift-left: _ -> [w5]
    stop <- "Stop" stop-if-true
    n2 = case shown="5" w11 {
      tunnel: [1 2 3 4 5 1] -> w10
      tunnel: [_ w34 w88 w129 w155 w176] -> w8
      tunnel: w7 -> [_ _ w90 w129 w155 w176]
      tunnel: [_ w40 _ _ _ _] -> w6
      tunnel: w5 -> [_ w35 _ _ _ _]
      tunnel: [_ w38 _ _ _ _] -> w4
      frame 0, Default {
        w16 = " " ("Befehl")
        w19 = "root" ("Username 2")
        # "State 0: Configure  RedPitaya"
        n3 = Current VI's Path() -> (path=w24:path)
        n4 = Strip Path(path=w24) -> (stripped path=w22:path)  [unwired: 1 out]
        n5 = Build Path(base path=w22, name or relative path="plink.exe" ("string")) -> (appended path=w21:path)
        n6 = Path To String(path=w21) -> (string=w18:string)
        n7 = Concatenate Strings(w18, w16, w19, "@" ("string"), "Host IP address", " -ssh", " -pw " ("string"), w19, w16, "-m " ("String"), "\"config.txt\"" ("String")) -> (w15:string)
        "Ausgeführter Befehl" <- w15
        n8 = call <vilib>:"System Exec.vi"("run minimized? (F)"=FALSE, "wait until completion? (T)"=FALSE, "standard input"=w15, "command line"=w15) -> ("standard error"=→"Fehlermeldung":string, "standard output"=→"Rückgabe":string)  [unwired: 2 in, 4 out]
        n9 = Wait (ms)(milliseconds to wait=u32 1000 ("Zu wartende ms")) -> ()  [unwired: 1 out]
      }
      frame 1 {
        # "Temp"
        # "Temp given as 10mV per °C"
        # "Temperature calculation"
        # "ADC offset"
        # "State 1: Signal Acquisition"
        n10 = local read "Host IP address"() -> (w33:string)
        n11 = TCP Open Connection(address=w33, remote port or service name=u16 5000, error in (no error)=w35) -> (connection ID=w37:refnum<k5>, error out=w36:errorcluster)  [unwired: 2 in]
        n12 = TCP Write(connection ID=w37, data in="ANALOG:PIN? AIN1\r\n" ("Verknüpfter String"), error in (no error)=w36, 9:"timeout ms (2000)") -> (connection ID out=w77:refnum<k5>, error out=w76:errorcluster)  [unwired: 1 out]
        n13 = TCP Read(connection ID=w77, bytes to read=524288 ("x*y"), error in (no error)=w76, 7:T2."CRLF" ("Modus (Standard)"), 9:"timeout ms (2000)") -> (connection ID out=w73:refnum<k5>, data out=w74:string, error out=w72:errorcluster)
        n14 = Fract/Exp String To Number(use system decimal point (T)=FALSE, string=w74) -> (number=w83:dbl)  [unwired: 2 in, 1 out]
        n15 = Subtract(x=w83, y=0.05) -> (x-y=w80:dbl)
        n16 = TCP Write(connection ID=w73, data in="ACQ:RST\r\nACQ:DEC 64;\r\nACQ:TRIG:DLY 8192;\r\nACQ:TRIG EXT_NE\r\nACQ:START\r\n" ("Verknüpfter String"), error in (no error)=w72, 9:"timeout ms (2000)") -> (connection ID out=w52:refnum<k5>, error out=w49:errorcluster)  [unwired: 1 out]
        n17 = for {
          N: 12 -> [_]
          tunnel: w52 -> [w87]
          tunnel: [w87] -> w51
          tunnel: w49 -> [w86]
          tunnel: [w86] -> w48
          n18 = Wait (ms)(milliseconds to wait=u32 10 ("Timer-Wert (ms)")) -> ()  [unwired: 1 out]
        }
        n19 = Multiply(x=w80, y=100.0) -> (x*y=→"Temp [°C]":dbl)
        n20 = TCP Write(connection ID=w51, data in="ACQ:DATA:FORMAT BIN\r\nACQ:SOUR1:DATA?\r\n" ("Verknüpfter String"), error in (no error)=w48, 9:"timeout ms (2000)") -> (connection ID out=w55:refnum<k5>, error out=w54:errorcluster)  [unwired: 1 out]
        n21 = TCP Read(connection ID=w55, bytes to read=2, error in (no error)=w54, 9:"timeout ms (2000)") -> (connection ID out=w66:refnum<k5>, data out=w62:string, error out=w65:errorcluster)  [unwired: 1 in]
        n22 = Divide(x=125000000.0, y=64.0) -> (x/y=→"Samplerate":dbl)
        n23 = Match Pattern(string=w62, regular expression="#") -> (after substring=w64:string)  [unwired: 1 in, 3 out]
        n24 = Decimal String To Number(string=w64) -> (number=w67:i32)  [unwired: 2 in, 1 out]
        n25 = TCP Read(connection ID=w66, bytes to read=w67, error in (no error)=w65, 9:"timeout ms (2000)") -> (connection ID out=w70:refnum<k5>, data out=w68:string, error out=w69:errorcluster)  [unwired: 1 in]
        n26 = Decimal String To Number(string=w68) -> (number=w71:i32)  [unwired: 2 in, 1 out]
        n27 = TCP Read(connection ID=w70, bytes to read=w71, error in (no error)=w69, 9:"timeout ms (2000)") -> (connection ID out=w47:refnum<k5>, data out=w59:string, error out=w46:errorcluster)  [unwired: 1 in]
        n28 = Unflatten From String(type=sgl[] [] ("Si"), binary string=w59, data includes array or string size? (T)=FALSE) -> (value=w34:sgl[])  [unwired: 2 in, 2 out]
        n29 = TCP Write(connection ID=w47, data in="ACQ:RST\r\n" ("Verknüpfter String"), error in (no error)=w46) -> (connection ID out=w40:refnum<k5>, error out=w38:errorcluster)  [unwired: 1 in, 1 out]
      }
      frame 2 {
        w102 = 1000 ("y")
        (unwired) 0.0 ("y")
        # "State 2: Segmentation"
        # "multiply by the\nspeed of sensor"
        # "divided by 2\n(reflected\nwave)"
        # "output/number of samples"
        # "8.389* min value\nof the peak"
        n30 = Array Size(array=w90) -> (size(s)=w93:i32)
        n31 = Add Array Elements(numeric array=w90) -> (sum=w94:sgl)
        n32 = Divide(x=w94, y=w93) -> (x/y=w92:sgl)
        n33 = Multiply(x=w92, y=sgl -1.0) -> (x*y=w89:sgl)
        n34 = Add(x=w90, y=w89) -> (x+y=w88:sgl[])
        "Sensor Signal" <- w88
        n35 = local read "Delay (# Samples)"() -> (w95:i32)
        n36 = call <vilib>:"Peak Detector.vi"("peaks/valleys"="Peaks/Valleys", "width"="Width", "threshold"="Peak Threshold", "X"=w88) -> ("Amplitudes"=→"Amplitude Peaks":dbl[], "Locations"=w125:dbl[], "# found"=→"Peaks Detected":i32)  [unwired: 3 in, 2 out]
        n37 = Subtract(x=w95, y=8192) -> (x-y=w106:i32)
        n38 = Threshold 1D Array(2:"Sample Threshold", 3:w125) -> (0:w128:dbl)  [unwired: 1 in]
        n39 = Round Toward +Infinity(x=w128) -> (ceil(x): smallest int >= x=w127:dbl)
        n40 = To Long Integer(number=w127) -> (32bit integer=w126:i32)
        n41 = Array Subset(array=w125, index=w126) -> (w110:dbl[])  [unwired: 1 in]
        "Location Peaks" <- w110
        n42 = Array Max & Min(array=w110) -> (min value=w107:dbl)  [unwired: 3 out]
        n43 = Array Subset(array=w88, index=3000 ("Index"), length=13384 ("Länge")) -> (w96:sgl[])
        n44 = Add(x=w107, y=w106) -> (x+y=w108:dbl)
        n45 = Array Max & Min(array=w96) -> (max index (indices)=w104:i32)  [unwired: 3 out]
        n46 = Multiply(x=0.008389, y=w108) -> (x*y=w123:dbl)
        n47 = Divide(x=w123, y=16384.0) -> (x/y=w121:dbl)
        n48 = Subtract(x=w104, y=w102) -> (x-y=w103:i32)
        n49 = Multiply(x=w102, y=2) -> (x*y=w100:i32)
        n50 = Divide(x=w121, y=2.0) -> (x/y=w119:dbl)
        n51 = Array Subset(array=w96, index=w103, length=w100) -> (→"Reflection":sgl[])
        n52 = Multiply(x=w119, y=33400.0) -> (x*y=→"Distance [cm]":dbl)
      }
      frame 3 {
        # "Peak\nDetection"
        # "Segmented Ultrasonic Signal"
        # "State 3: Feature Extraction 1"
        n53 = xnode "Spektrum ermitteln"("Signale"=w129) -> ("FFT - (RMS)"=w132:cluster{"f0":dbl, "df":dbl, "magnitude":dbl[]})  [unwired: 1 in, 2 out]
        "Fourier Spectrum" <- w132
        n54 = Unbundle(w132) -> ("magnitude"=w141:dbl[])  [unwired: 2 out]
        n55 = call "In dynamische Daten konvertieren"("Array"=w129) -> ("Dynamic Data Type"=w139:dynamicdata)  [unwired: 3 in]
        n56 = call "Verzerrungsmessung"("Signals"=w139) -> ("SINAD (dB)"=→"SINAD (dB)":dynamicdata)  [unwired: 9 in, 1 out]
        n57 = Array Subset(array=w141, index=160, length=22 ("Länge")) -> (w134:dbl[])
        n58 = call <vilib>:"Peak Detector.vi"("width"="Width peak detect.", "threshold"="Threshold peak detect.", "X"=w134) -> ("Locations"=w135:dbl[], "# found"=→"# Peaks":i32)  [unwired: 4 in, 3 out]
        n59 = Index Array(array=w135, index=0 ("Index")) -> (element=→"Loc 1st Peak":dbl)
      }
      frame 4 {
        # "State 4: Feature Extraction 2"
        n60 = call "Convert to Dynamic Data"("Array"=w155) -> ("Dynamic Data Type"=w154:dynamicdata)  [unwired: 3 in]
        n61 = call "Amplitude and Level Measurements"("Signals"=w154) -> ("Mean (DC)"=→"Mean (DC)":dynamicdata, "RMS"=→"RMS Value":dynamicdata, "Negative Peak"=→"Negative Peak":dynamicdata, "Positive Peak"=→"Positive Peak":dynamicdata, "Peak to Peak"=→"Peak to Peak":dynamicdata)  [unwired: 9 in, 1 out]
      }
      frame 5 {
        # "State 5: Machine Decision Making / Machine Learning"
        n62 = Current VI's Path() -> (path=w166:path)
        n63 = Strip Path(path=w166) -> (stripped path=w163:path)  [unwired: 1 out]
        n64 = Open Python Session(python version="3.6" ("Python version")) -> (session out=w175:refnum<k35>, error out=w174:errorcluster)  [unwired: 2 in]
        n65 = Build Path(base path=w163, name or relative path=path "Project.py" ("module path")) -> (appended path=w164:path)
        n66 = node "Python Node"(w175, w164, "classifier" ("function name"), w174, "Number 1", "Number 1", "Number 2") -> (w173:refnum<k35>, w172:errorcluster, →"Result":dbl)  [unwired: 2 in, 2 out]
        n67 = Close Python Session(session in=w173, error in=w172) -> (11:→"error out 2":errorcluster)
      }
    }
  }
  n68 = TCP Close Connection(connection ID=w2, error in (no error)=w1) -> ()  [unwired: 1 in, 2 out]
